vi "UE9 eDI Example.vi"() -> (0 "error out":errorcluster)   [LabVIEW 2021]
panel:
  in  "Address":string="192.168.1.209"
  in  "ConnectionType":u16(ring) items=["LJ_ctUSB", "LJ_ctETHERNET"]
  in  "FirstFound":bool=TRUE
  out "State":bool
  in  "Channel":i32
  out "Error Message":string
  # "Reads 1 digital input using the UD easy function eDI."
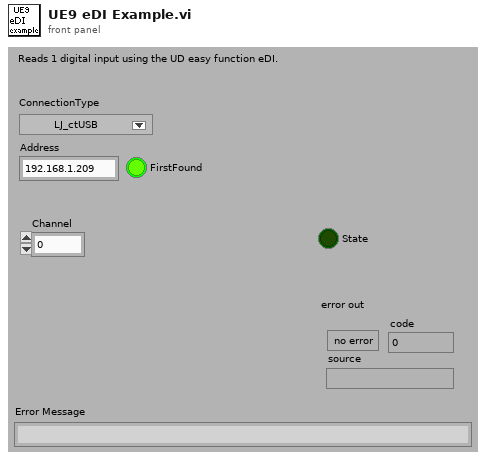
[diagram p1: front panel]
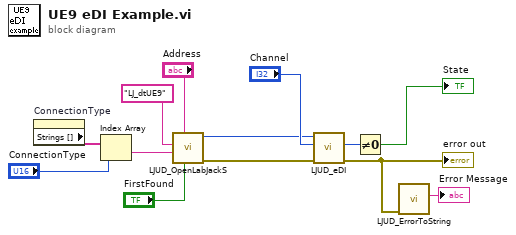
[diagram p0: block diagram]
diagram:
  n1 = property on="ConnectionType" class="Ring (strict)"() -> ("Strings []"=w8:string[])  [unwired: 2 in, 2 out]
  n2 = Index Array(array=w8, index="ConnectionType") -> (element=w4:string)
  n3 = call "LJUD_OpenLabJackS.vi"("FirstFound"="FirstFound", "Address"="Address", "ConnectionType"=w4, "DeviceType"="LJ_dtUE9") -> ("error out"=w1:errorcluster, "Handle"=w2:i32)  [unwired: 5 in, 1 out]
  n4 = call "LJUD_eDI.vi"("error in"=w1, "Channel"="Channel", "Handle In"=w2) -> ("error out"=w12:errorcluster, "State"=w10:i32)  [unwired: 6 in, 1 out]
  "error out" <- w12
  n5 = Not Equal To 0?(x=w10) -> (x != 0?=→"State":bool)
  n6 = call "LJUD_ErrorToString.vi"("error in"=w12) -> ("String"=→"Error Message":string)  [unwired: 10 in]
